vi "Read_TPG300_sensor (SubVI).vi"(7 "Sensor CMD":string, 8 "error in (no error)":errorcluster, 11 "TCP Network Connection in":refnum<k5>) -> (0 "error out":errorcluster, 3 "connection ID out":refnum<k5>, 4 "out number":dbl, 5 "data out":string)   [LabVIEW 2013]
uses:
  <vilib>/Utility/error.llb/DialogType.ctl
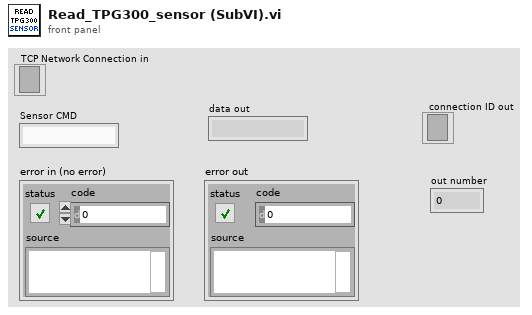
[diagram p1: front panel]
types:
  T1 = typedef "DialogType.ctl" = u16
  T2 = enum16{"Standard", "Buffered", "CRLF", "Immediate"}
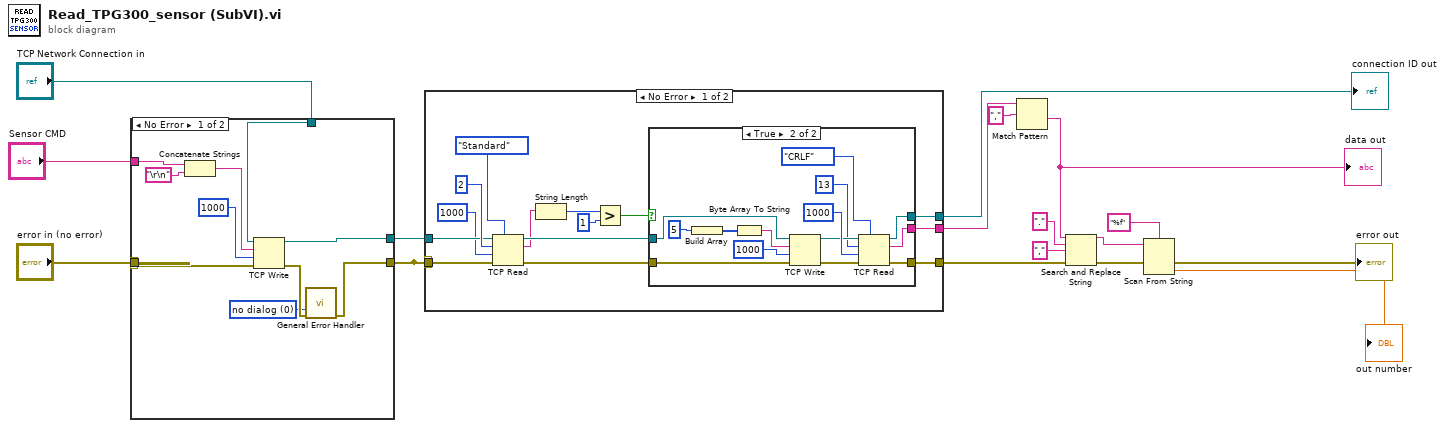
[diagram p0: block diagram]
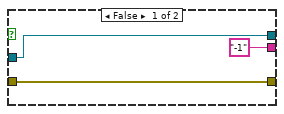
[diagram p2: hidden frame]
diagram:
  n1 = case shown="No Error" "error in (no error)" {
    tunnel: [w19 w29] -> w3
    tunnel: [w27 w28] -> w17
    tunnel: "Sensor CMD" -> [w24 _]
    tunnel: "TCP Network Connection in" -> [w22 w28]
    tunnel: "error in (no error)" -> [w21 w29]
    frame No Error {
      w18 = T1 0 items=["no dialog", "OK message", "continue or stop message", "OK message + warnings", "continue/stop + warnings"] ("type of dialog (OK msg:1)")
      n2 = Concatenate Strings(w24, "\r\n") -> (w25:string)
      n3 = TCP Write(connection ID=w22, data in=w25, error in (no error)=w21, 9:1000 ("timeout ms (25000)")) -> (connection ID out=w27:refnum<k5>, error out=w20:errorcluster)  [unwired: 1 out]
      n4 = call <vilib>:"General Error Handler.vi"("type of dialog (OK msg:1)"=w18, "error in (no error)"=w20) -> ("error out"=w19:errorcluster)  [unwired: 9 in, 4 out]
    }
    frame Error {
    }
  }
  n5 = case shown="No Error" w3 {
    tunnel: w3 -> [w36 w61]
    tunnel: w17 -> [w35 w62]
    tunnel: [w32 w62] -> w15
    tunnel: [w31 _] -> w9
    tunnel: [w30 w61] -> w8
    frame No Error {
      n6 = TCP Read(connection ID=w35, bytes to read=2, error in (no error)=w36, 7:T2."Standard" ("mode (standard)"), 9:1000 ("timeout ms (25000)")) -> (connection ID out=w39:refnum<k5>, data out=w37:string, error out=w38:errorcluster)
      n7 = String Length(string=w37) -> (length=w41:i32)
      n8 = Greater?(x=w41, y=1) -> (0:w43:bool)
      n9 = case shown="True" w43 {
        tunnel: [w46 w60] -> w30
        tunnel: ["-1" ("data out") w51] -> w31
        tunnel: w38 -> [w46 w50]
        tunnel: w39 -> [w45 w49]
        tunnel: [w45 w47] -> w32
        frame False {
        }
        frame True {
          n10 = Build Array(u8 5 ("millisecond multiple")) -> (w57:u8[])
          n11 = Byte Array To String(unsigned byte array=w57) -> (string=w56:string)
          n12 = TCP Write(connection ID=w49, data in=w56, error in (no error)=w50, 9:1000 ("timeout ms (25000)")) -> (connection ID out=w52:refnum<k5>, error out=w53:errorcluster)  [unwired: 1 out]
          n13 = TCP Read(connection ID=w52, bytes to read=13 ("timeout ms (25000)"), error in (no error)=w53, 7:T2."CRLF" ("mode (standard)"), 9:1000 ("timeout ms (25000)")) -> (connection ID out=w47:refnum<k5>, data out=w51:string, error out=w60:errorcluster)
        }
      }
    }
    frame Error {
    }
  }
  "connection ID out" <- w15
  n14 = Match Pattern(string=w9, regular expression=",") -> (after substring=w4:string)  [unwired: 1 in, 3 out]
  "data out" <- w4
  n15 = Search and Replace String(input string=w4, search string=".", replace string="," ("replace string (\"\")"), error in=w8) -> (result string=w14:string, error out=w7:errorcluster)  [unwired: 4 in, 2 out]
  n16 = Scan From String(format string="%f", input string=w14, error in=w7) -> (error out=→"error out":errorcluster, output 1=→"out number":dbl)  [unwired: 2 in, 2 out]
